vi "Update ROI waveform cursor snap selector.vi"(4 "Reset selection to the first element":bool, 8 "error in (no error)":errorcluster, 11 "Sorted Pointers":i32[](array[numeric])) -> (0 "error out":errorcluster)   [LabVIEW 2013]
uses:
  Global variables/gl_Functional Imaging-Global variables.vi
  Program Files (x86)/National Instruments/LabVIEW 2013/user.lib/_OpenG.lib/array/array.llb/Reorder 1D Array2 (String)__ogtk.vi
  Program Files (x86)/National Instruments/LabVIEW 2013/user.lib/_OpenG.lib/array/array.llb/Reorder 1D Array2 (Boolean)__ogtk.vi
  Program Files (x86)/National Instruments/LabVIEW 2013/user.lib/_OpenG.lib/array/array.llb/Search 1D Array (Boolean)__ogtk.vi
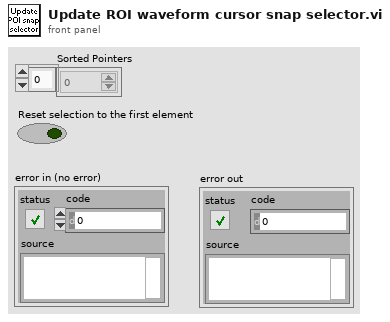
[diagram p1: front panel]
types:
  T1 = typedef "Functional Imging UI Refs.ctl" = cluster{"Menu ref":refnum<k9>, "Image control":refnum<vi>, "VI ref":refnum<vi>, "XGrapher":refnum<vi>, "Smoothing":refnum<vi>, "POI Averaging":refnum<vi>, "Normalize":refnum<vi>, "POI data points in each trial":refnum<vi>, "Channel":refnum<vi>, "Experiment data folder path":refnum<vi>, "[ROI vis]":refnum<vi>, "[Groups] visbl":T2, "Group Name":refnum<vi>, "POI index":refnum<vi>, "Trial No.":refnum<vi>, "Intensity Zoom":refnum<vi>, "Trial Cursor Enabled":refnum<vi>, "Number of Trials (ind 1)":refnum<vi>, "Number of Trials (ind 2)":refnum<vi>, "MiniScans Available":refnum<vi>, "POI Available":refnum<vi>, "Defer graph updates":refnum<vi>, "Waveform selector":refnum<vi>, "#of selected POI":refnum<vi>, "#of selected MiniScans":refnum<vi>, "#of selected groups":refnum<vi>, "Max Z-Projection":refnum<vi>, "Z-Plane Selector":refnum<vi>, "Index of miniscan point to visualise":refnum<vi>, "ROI vis. mode":refnum<vi>, "Total # of points":refnum<vi>, "Index of group clicked on":refnum<vi>, "Pane 1":refnum<vi>, "Pane 2":refnum<vi>, "Pane 3":refnum<vi>, "Pane 4":refnum<vi>, "Pane 5":refnum<vi>, "Pane 6":refnum<vi>, "Deselect all ROI":refnum<vi>, "Deselect all groups":refnum<vi>}
  T2 = typedef "Groups array referecne.ctl" = refnum<vi>
  T3 = typedef "ROI selector array.ctl" = T4[]
  T4 = typedef "Interface-ROI selection cluster.ctl" = cluster{"ROI number":i32, "ROI ID":T5, "Visibility":bool}
  T5 = typedef "ROI ID Enum.ctl" = enum16{"Point", "MiniScan", "Comp. MiniScan", "Rectangle", "Comp. volume", "Arb. plane point"}
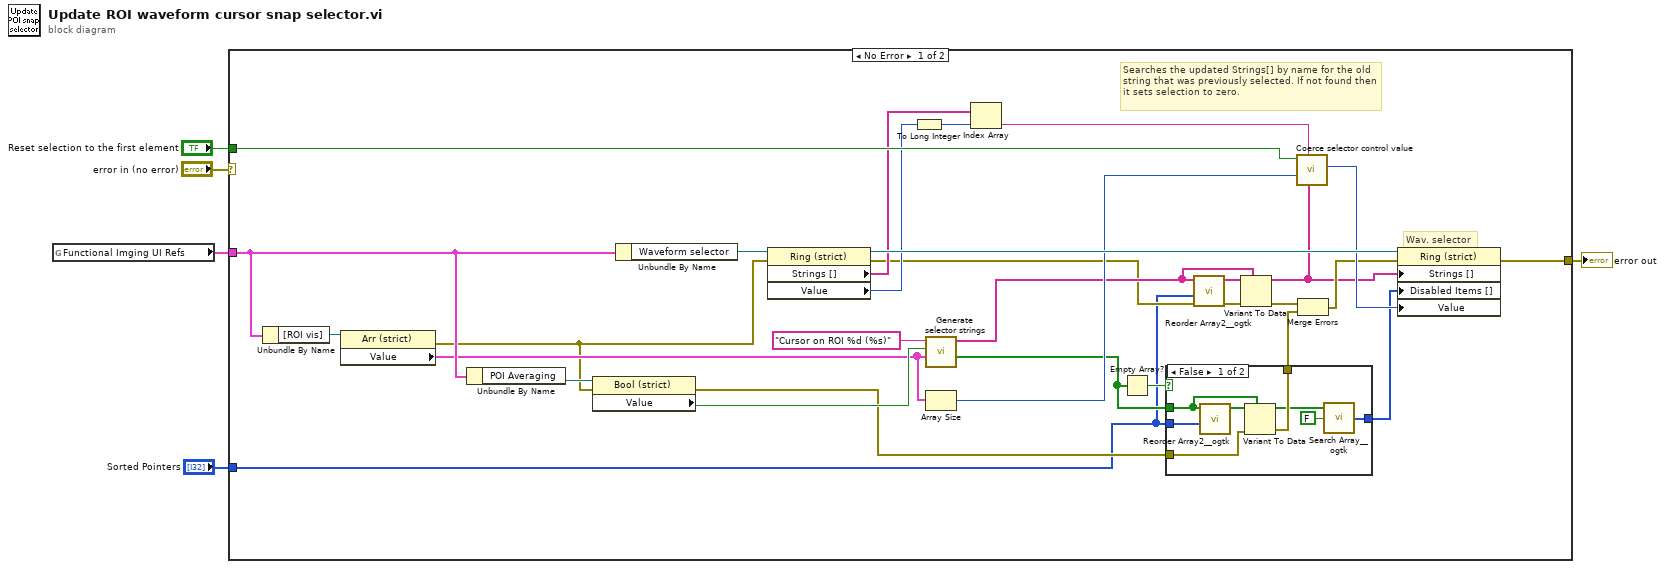
[diagram p0: block diagram]
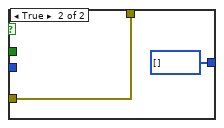
[diagram p2: hidden frame]
diagram:
  n1 = global read "gl_Functional Imaging-Global variables.vi" "Functional Imging UI Refs"() -> (w2:T1)
  n2 = case shown="No Error" "error in (no error)" {
    selector: "error in (no error)" -> [_ w45]
    tunnel: [w9 w45] -> w5
    tunnel: w2 -> [w20 _]
    tunnel: "Reset selection to the first element" -> [w19 _]
    tunnel: "Sorted Pointers" -> [w6 _]
    frame No Error {
      # "Searches the updated Strings[] by name for the old string that was previously selected. If not found then it sets selection to zero."
      # "Wav. selector"
      # "Updates the POI waveform selector control"
      n3 = Unbundle By Name(w20) -> ("[ROI vis]"=w21:refnum<vi>)
      n4 = property on="Property Node" class="Arr (strict)"(reference=w21) -> (error out=w7:errorcluster, "Value"=w18:T3)  [unwired: 1 in, 1 out]
      n5 = Unbundle By Name(w20) -> ("POI Averaging"=w31:refnum<vi>)
      n6 = property on="Property Node" class="Bool (strict)"(reference=w31, error in=w7) -> (error out=w17:errorcluster, "Value"=w30:bool)  [unwired: 1 out]
      n7 = Unbundle By Name(w20) -> ("Waveform selector"=w33:refnum<vi>)
      n8 = property on="Property Node" class="Ring (strict)"(reference=w33, error in=w7) -> (reference out=w34:refnum<vi>, error out=w8:errorcluster, "Strings []"=w16:string[], "Value"=w15:u16)
      n9 = To Long Integer(number=w15) -> (32bit integer=w14:i32)
      n10 = call "Generate selector strings.vi"("[POI#] or [MiniScan#]"=w18, "POI Averaged"=w30, "format string"="Cursor on ROI %d (%s)") -> ("[Visibility]"=w10:bool[], "Strings[]"=w11:string[])  [unwired: 7 in]
      n11 = Array Size(array=w18) -> (size(s)=w29:i32)
      n12 = Index Array(array=w16, index=w14) -> (element=w13:string)
      n13 = Empty Array?(array=w10) -> (empty?=w23:bool)
      n14 = case shown="False" w23 {
        tunnel: w6 -> [w41 _]
        tunnel: [w35 i32[] [] ("Indices of Elements")] -> w22
        tunnel: w10 -> [w40 _]
        tunnel: [w39 w44] -> w26
        tunnel: w17 -> [w38 w44]
        frame False {
          n15 = call-poly "Reorder Array2__ogtk.vi"("indices"=w41, "array"=w40) -> ("reordered array"=w42:bool[])  [unwired: 9 in]
          n16 = Variant To Data(error in=w38, type=w40, Variant=w42) -> (data=w36:bool[], error out=w39:errorcluster)
          n17 = call-poly "Search Array__ogtk.vi"("Array"=w36, "Element Data"=FALSE) -> ("Indices of Elements"=w35:i32[])  [unwired: 7 in]
        }
        frame True {
        }
      }
      n18 = call-poly "Reorder Array2__ogtk.vi"("indices"=w6, "array"=w11) -> ("reordered array"=w27:string[])  [unwired: 9 in]
      n19 = Variant To Data(error in=w8, type=w11, Variant=w27) -> (data=w12:string[], error out=w25:errorcluster)
      n20 = call "Coerce selector control value.vi"("New strings[]"=w12, "String of currently selected item"=w13, "#of selected ROI"=w29, "Set selection to index 0"=w19) -> ("Selection index out"=w28:u16)  [unwired: 7 in]
      n21 = Merge Errors(w25, w26) -> (w24:errorcluster)
      n22 = property on="Property Node" class="Ring (strict)"(reference=w34, error in=w24, "Strings []"=w12, "Disabled Items []"=w22, "Value"=w28) -> (error out=w9:errorcluster)  [unwired: 1 out]
    }
    frame Error {
    }
  }
  "error out" <- w5
